vi "Get Pathloss Data.vi"() -> ()   [LabVIEW 2011]
panel:
  out "External Attenuation, dB":dbl format="%.2f"
  in  "Folder Path":path=path "C:/LVProject_Dll/WLAN Reference/System Calibration"
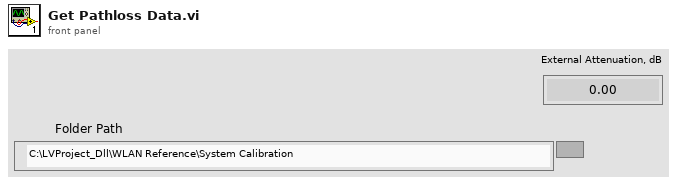
[diagram p1: front panel]
types:
  T1 = cluster{"Temperature, C":dbl, "Time Stamp, sec":dbl, "Calibration Table":dbl[][]}
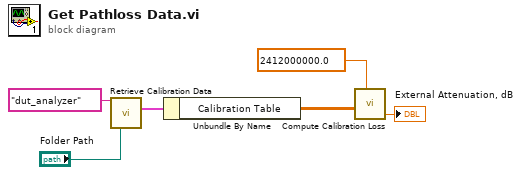
[diagram p0: block diagram]
diagram:
  n1 = call "Retrieve Calibration Data.vi"("Calibration Signal Path Name"="dut_analyzer", "Folder Path"="Folder Path") -> ("Calibration Data"=w6:T1)  [unwired: 12 in, 1 out]
  n2 = Unbundle By Name(w6) -> ("Calibration Table"=w5:dbl[][])
  n3 = call "Compute Calibration Loss.vi"("Table (frequency, power, pathloss)"=w5, "Center Frequency, Hz"=2412000000.0) -> ("External Attenuation, dB"=→"External Attenuation, dB":dbl)  [unwired: 3 in, 2 out]
